vi "Result.Build Measurement Result Item.vi"(4 "AddDesc":string, 5 "Error=>Fail":bool, 6 "ForceFail":bool, 7 "Log(F)/Pass(T)":bool, 8 "Error In(Result Error)":errorcluster, 9 "Value":string, 10 "Name":string, 11 "Category":string) -> (0 "Error Out(No Error)":errorcluster, 2 "Fail/Error":bool, 3 "Meas":T1 {"Status" items=["LOG", "PASS", "FAIL", "ERROR"]})   [LabVIEW 2024]
uses:
  Result.Measurement Item.ctl
  Result.Measurement and Attribute Item Status.ctl
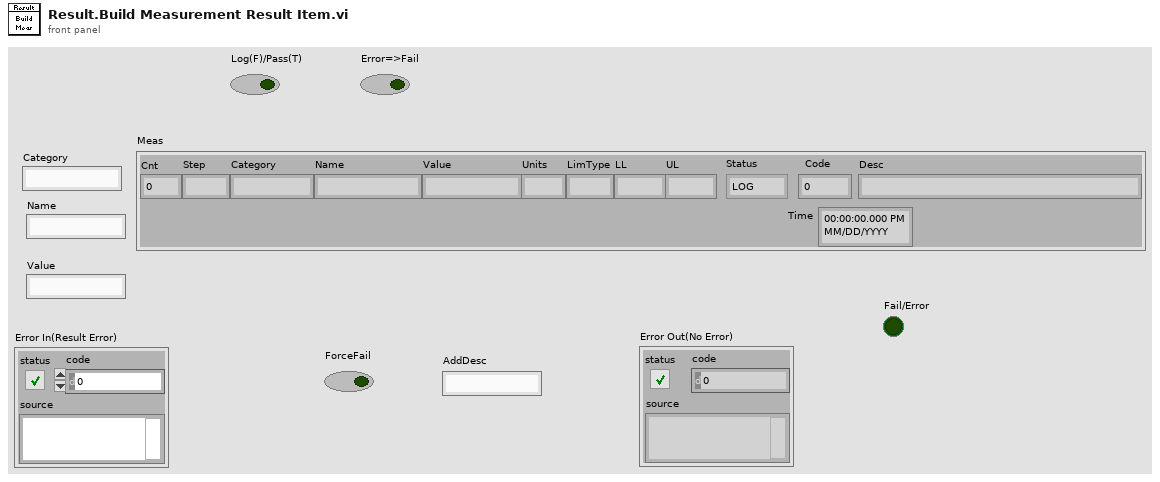
[diagram p1: front panel]
types:
  T1 = typedef "Result.Measurement Item.ctl" = cluster{"Cnt":i32, "Step":string, "Category":string, "Name":string, "Value":string, "Units":string, "LimType":string, "LL":string, "UL":string, "Status":T2, "Code":i32, "Desc":string, "Time":timestamp}
  T2 = typedef "Result.Measurement and Attribute Item Status.ctl" = i32
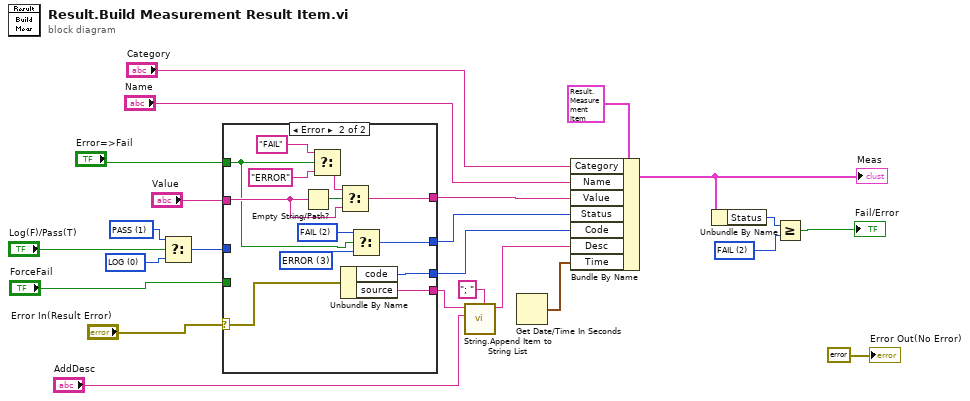
[diagram p0: block diagram]
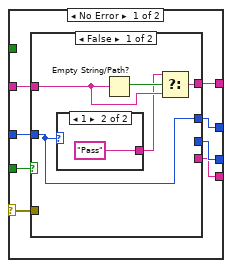
[diagram p2: hidden frame]
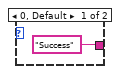
[diagram p3: hidden frame]
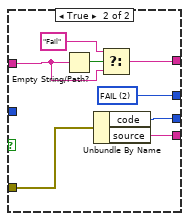
[diagram p4: hidden frame]
diagram:
  w14 = T2 1 items=["LOG", "PASS", "FAIL", "ERROR"] ("Status")
  w13 = T2 0 items=["LOG", "PASS", "FAIL", "ERROR"] ("Status")
  w19 = T2 2 items=["LOG", "PASS", "FAIL", "ERROR"] ("y")
  n1 = Select(t=w14, s="Log(F)/Pass(T)", f=w13) -> (s? t:f=w11:T2)
  n2 = case shown="Error" "Error In(Result Error)" {
    selector: "Error In(Result Error)" -> [w25 w56]
    tunnel: "ForceFail" -> [w32 _]
    tunnel: [w31 w49] -> w16
    tunnel: [w30 w58] -> w15
    tunnel: [w29 w57] -> w5
    tunnel: w11 -> [w28 _]
    tunnel: "Value" -> [w27 w55]
    tunnel: [w26 w59] -> w8
    tunnel: "Error=>Fail" -> [_ w48]
    frame No Error {
      n3 = case shown="False" w32 {
        tunnel: [w34 w47] -> w31
        tunnel: w25 -> [_ w46]
        tunnel: [_ w45] -> w30
        tunnel: [_ w44] -> w29
        tunnel: w28 -> [w34 _]
        tunnel: w27 -> [w35 w42]
        tunnel: [w36 w40] -> w26
        frame False {
          n4 = case shown="1" w34 {
            tunnel: ["Success" "Pass"] -> w33
            frame 0, Default {
            }
            frame 1 {
            }
          }
          n5 = Empty String/Path?(string/path=w35) -> (empty?=w37:bool)
          n6 = Select(t=w33, s=w37, f=w35) -> (s? t:f=w36:string)
        }
        frame True {
          w47 = T2 2 items=["LOG", "PASS", "FAIL", "ERROR"] ("Status")
          n7 = Empty String/Path?(string/path=w42) -> (empty?=w43:bool)
          n8 = Unbundle By Name(w46) -> ("code"=w45:i32, "source"=w44:string)
          n9 = Select(t="Fail", s=w43, f=w42) -> (s? t:f=w40:string)
        }
      }
    }
    frame Error {
      w50 = T2 2 items=["LOG", "PASS", "FAIL", "ERROR"] ("Status")
      w51 = T2 3 items=["LOG", "PASS", "FAIL", "ERROR"] ("Status")
      n10 = Empty String/Path?(string/path=w55) -> (empty?=w60:bool)
      n11 = Select(t="FAIL", s=w48, f="ERROR") -> (s? t:f=w52:string)
      n12 = Select(t=w52, s=w60, f=w55) -> (s? t:f=w59:string)
      n13 = Unbundle By Name(w56) -> ("code"=w58:i32, "source"=w57:string)
      n14 = Select(t=w50, s=w48, f=w51) -> (s? t:f=w49:T2)
    }
  }
  n15 = call "String.Append Item to String List.vi"("Delimiter"="; ", "New Data"="AddDesc", "Existing Str"=w5) -> ("New Str"=w3:string)  [unwired: 8 in]
  n16 = Get Date/Time In Seconds() -> (seconds since 1Jan1904=w6:timestamp)
  n17 = Bundle By Name(cluster=T1 {"Cnt"=0, "Step"="", "Category"="", "Name"="", "Value"="", "Units"="", "LimType"="", "LL"="", "UL"="", "Status"=0, "Code"=0, "Desc"="", "Time"=timestamp(0 s since 1904-01-01)} ("Meas"), "Category"="Category", "Name"="Name", "Value"=w8, "Status"=w16, "Code"=w15, "Desc"=w3, "Time"=w6) -> (w10:T1)
  "Meas" <- w10
  n18 = Unbundle By Name(w10) -> ("Status"=w20:T2)
  n19 = Greater Or Equal?(x=w20, y=w19) -> (x >= y?=→"Fail/Error":bool)
  "Error Out(No Error)" <- errorcluster {"status"=FALSE, "code"=0, "source"=""} ("Error Out(No Error)")
